vi "Module Init.vi"(8 "error in (no error)":errorcluster, 11 "Event Viewer Module in":refnum<class "Event Viewer Module.lvclass">) -> (0 "error out":errorcluster, 3 "Event Viewer Module out":refnum<class "Event Viewer Module.lvclass">)   [LabVIEW 2020, in "VolatusGUI.lvlib" / "Event Viewer Module.lvclass"]
uses:
  Event Viewer Module.lvclass
  C:/dev/lv20CE/relink/lv-volatus/Volatus/Module/Module.lvclass
  Event Element.ctl
  Event Viewer Module.lvclass/Event Viewer Module.ctl
  Volatus/Module/Module.lvclass/Module.ctl
  Volatus/MessageQ/MessageQ.lvclass/MessageQ.ctl
  Volatus/Module/Self Q.vi
  Volatus/MessageQ/Send.vi
  Volatus/Module/Module.lvclass
  C:/dev/lv20CE/relink/lv-volatus/VolatusGUI/Event Viewer Module/Event Viewer Module.lvclass
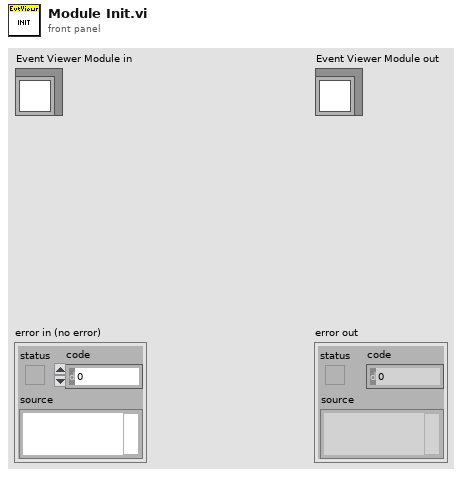
[diagram p1: front panel]
types:
  T1 = typedef "VolatusGUI.lvlib/Event Viewer Module.lvclass/Event Element.ctl" = cluster{"Node":string, "Node Color":u32, "Timestamp":string, "TS Color":u32, "Level":string, "Level Color":u32, "Context":string, "Context Color":u32, "Message":string, "Error Code":i32, "Error Source":string}
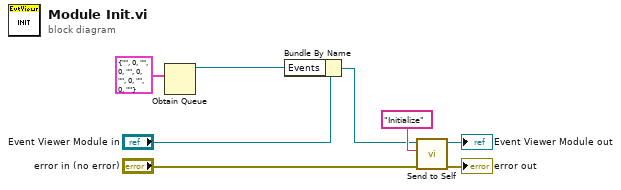
[diagram p0: block diagram]
diagram:
  n1 = Obtain Queue(element data type=T1 {"Node"="", "Node Color"=0, "Timestamp"="", "TS Color"=0, "Level"="", "Level Color"=0, "Context"="", "Context Color"=0, "Message"="", "Error Code"=0, "Error Source"=""} ("Event Element")) -> (queue out=w1:refnum<queue>)  [unwired: 4 in, 2 out]
  n2 = Bundle By Name(cluster="Event Viewer Module in", "Events"=w1) -> (w2:refnum<class "Event Viewer Module.lvclass">)
  n3 = call "Send to Self.vi"("error in (no error)"="error in (no error)", "Message ID"="Initialize", "Module in"=w2) -> ("error out"=→"error out":errorcluster, "Module in"=→"Event Viewer Module out":refnum<class "Event Viewer Module.lvclass">)  [unwired: 7 in]
